vi "removePage.vi"(8 "error in (no error)":errorcluster, 10 "Page Name":string, 11 "MS-Excel in":refnum<class "MS-Excel.lvclass">) -> (0 "error out":errorcluster, 3 "MS-Excel out":refnum<class "MS-Excel.lvclass">)   [LabVIEW 2017, in "LabVIEW NPOI.lvlib" / "MS-Excel.lvclass"]
uses:
  MS-Excel.lvclass
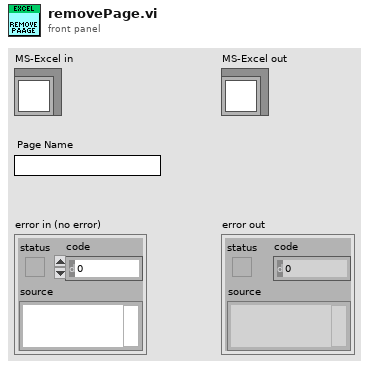
[diagram p1: front panel]
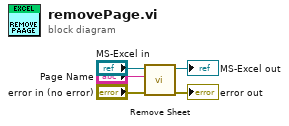
[diagram p0: block diagram]
diagram:
  n1 = call "Remove Sheet.vi"("error in (no error)"="error in (no error)", "Sheet Name"="Page Name", "MS-Excel in"="MS-Excel in") -> ("error out"=→"error out":errorcluster, "MS-Excel out"=→"MS-Excel out":refnum<class "MS-Excel.lvclass">)  [unwired: 7 in]
